vi "AlGaInPAs_Layer.vi"(0 "Al run":bool, 1 "Al Flow":dbl, 2 "In run":bool, 3 "Ga run":bool, 4 "Ga Flow":dbl, 5 "PH3 run":bool, 6 "PH3 Flow":dbl, 7 "In Flow":dbl, 8 "AsH3 run":bool, 9 "AsH3 Flow":dbl) -> ()   [LabVIEW 2011]
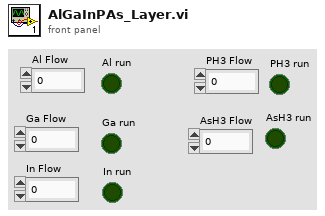
[diagram p1: front panel]
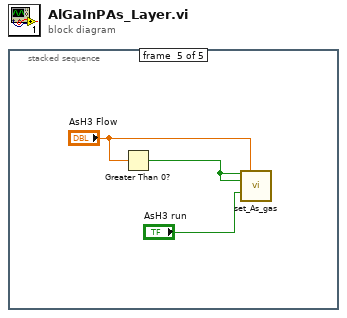
[diagram p0: block diagram]
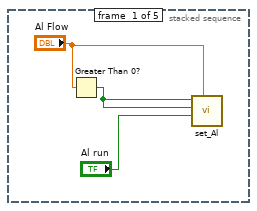
[diagram p2: hidden frame]
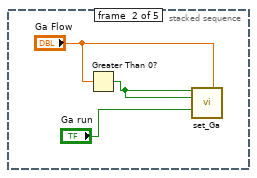
[diagram p3: hidden frame]
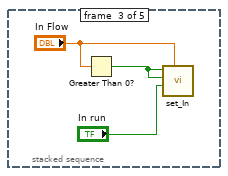
[diagram p4: hidden frame]
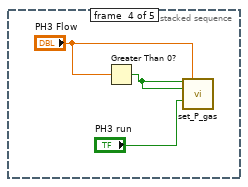
[diagram p5: hidden frame]
diagram:
  n1 = stacked-sequence {
    frame #0 {
      n2 = Greater Than 0?(x="Al Flow") -> (x > 0?=w1:bool)
      n3 = call "set_Al.vi"("Aluminum Flow"="Al Flow", "Al Run"="Al run", "Al Bubbler"=w1, "Al Active"=w1) -> ()  [unwired: 6 in]
    }
    frame #1 {
      n4 = Greater Than 0?(x="Ga Flow") -> (x > 0?=w4:bool)
      n5 = call "set_Ga.vi"("Ga Active"=w4, "Ga Flow 1"="Ga Flow", "Ga Bubbler"=w4, "Ga Run"="Ga run") -> ()  [unwired: 4 in, 8 out]
    }
    frame #2 {
      n6 = Greater Than 0?(x="In Flow") -> (x > 0?=w7:bool)
      n7 = call "set_In.vi"("Indium Flow"="In Flow", "In Run"="In run", "In Bubbler"=w7, "In Active"=w7) -> ()  [unwired: 1 in, 5 out]
    }
    frame #3 {
      n8 = Greater Than 0?(x="PH3 Flow") -> (x > 0?=w10:bool)
      n9 = call "set_P_gas.vi"("P_Gas Active"=w10, "P_Gas Flow"="PH3 Flow", "P_Gas In"=w10, "P_Gas Run"="PH3 run") -> ()  [unwired: 2 in, 10 out]
    }
    frame #4 {
      n10 = Greater Than 0?(x="AsH3 Flow") -> (x > 0?=w13:bool)
      n11 = call "set_As_gas.vi"("As_Gas Active"=w13, "As_Gas Flow"="AsH3 Flow", "As_Gas In"=w13, "As_Gas Run"="AsH3 run") -> ()  [unwired: 2 in, 10 out]
    }
  }
